vi "pipe writer.vi"() -> ()   [LabVIEW 2013, in "Unix Pipes.lvlib"]
uses:
  Unix Pipes.lvlib
  <vilib>/Platform/TimedLoop/XDataNode/timing_clust.ctl
  <vilib>/Platform/TimedLoop/XDataNode/nitl_modes.ctl
  <vilib>/Platform/TimedLoop/XDataNode/wakeup.ctl
  Classes/Unix Pipe Writer/Open Pipe (writer).vi
  Classes/Unix Pipe Writer/Close Pipe (writer).vi
  <vilib>/NI/NI Linux RT Utilities/VIs/Public/Time/Get Clock Time (timespec).vi
  <vilib>/platform/TimedLoop/XDataNode/XDataNode.xnode
  <vilib>/NI/NI Linux RT Utilities/Linux RT Utilities.lvlib
  Classes/Unix Pipe Writer/Unix Pipe Writer.lvclass
  <vilib>/Platform/TimedLoop/XDataNode/XDNodeRunTimeDep.lvlib
panel:
  out "pipe already exists?":bool
  in  "stop":bool
  out "time":cluster{"sec":u64, "nsec":u64}
  out "error out":errorcluster
  out "bytes written":i32
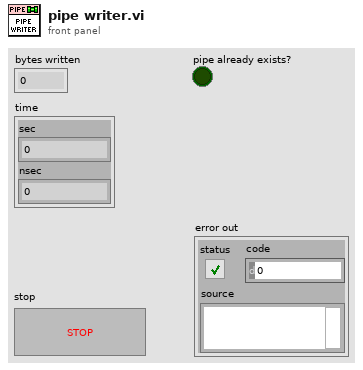
[diagram p1: front panel]
types:
  T1 = typedef "XDNodeRunTimeDep.lvlib/timing_clust.ctl" = cluster{"Expected End [f-1]":u64, "Actual End [f-1]":u64, "Finished Late? [f-1]":bool, "Expected End [i-1]":u64, "Actual End [i-1]":u64, "Finished Late? [i-1]":bool, "Expected Start [i]":u64, "Actual Start [i]":u64, "Expected Start [f]":u64, "Actual Start [f]":u64, "Source Name":string, "Structure Name":string, "Period":i64, "Deadline":i64, "Offset":i64, "Start":i64, "Priority":i32, "Timeout":i32, "Mode":T2, "Wakeup Reason":T3, "Error":errorcluster, "Source Type":string, "Secondary Source Type":string, "Global End Time":u64, "Global Start Time":u64, "Frame Duration":u64, "Iteration Duration":u64, "Assigned CPU":i32, "I/O Scan Engine Mode":u32}
  T2 = typedef "XDNodeRunTimeDep.lvlib/nitl_modes.ctl" = enum32{"No Change", "Process missed periods, maintain original phase", "Discard missed periods, maintain original phase", "Process missed periods, ignore original phase", "Discard missed periods, ignore original phase"}
  T3 = typedef "XDNodeRunTimeDep.lvlib/wakeup.ctl" = enum32{"Normal", "Aborted", "Asynchronous wakeup", "Timing source error", "Timed loop error", "Timeout"}
  T4 = enum16{"big-endian, network order", "native, host order", "little-endian"}
  T5 = cluster{"Stop":bool, "Time":cluster{"sec":u64, "nsec":u64}}
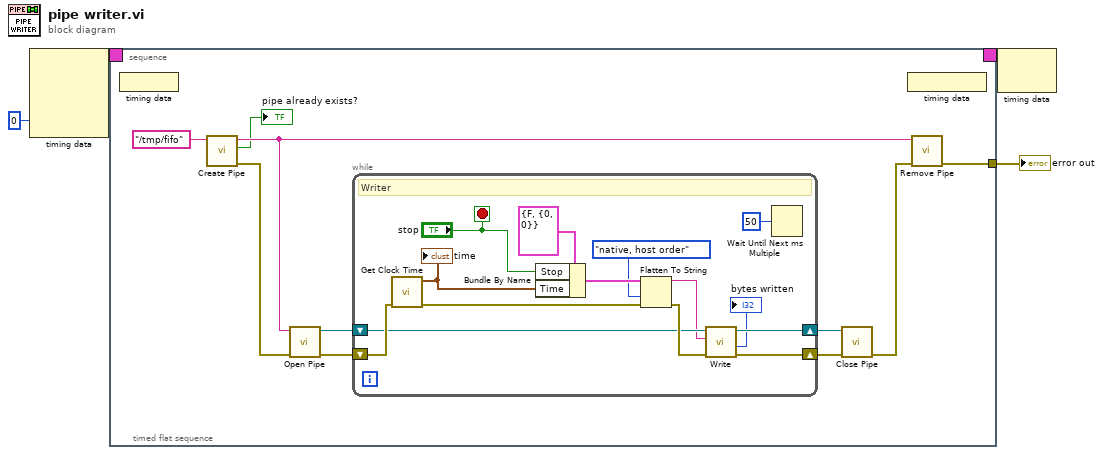
[diagram p0: block diagram]
diagram:
  n1 = node-c288(0 ("Processor")) -> (w3:T1)  [unwired: 3 in]
  n2 = timed-sequence {
    timing: w3 -> [_]
    timing-out: [_] -> w2
    tunnel: [w5] -> w4
    n3 = timed-flat-sequence {
      tunnel: [w13] -> w5
      n4 = node-c288() -> ()  [unwired: 1 in]
      n5 = call "Create Pipe.vi"("pathname in"="/tmp/fifo") -> ("error out"=w14:errorcluster, "pipe already exists?"=→"pipe already exists?":bool, "pathname out"=w7:string)  [unwired: 8 in]
      n6 = call-poly "Open Pipe.vi"("error in (no error)"=w14, "pathname in"=w7) -> ("error out"=w8:errorcluster, "pipe writer out"=w12:refnum<data-value>)  [unwired: 8 in]
      n7 = while {
        shift-right: [w28] -> w11
        shift-left: w12 -> [w17]
        shift-right: [w27] -> w10
        shift-left: w8 -> [w25]
        stop <- "stop" stop-if-true
        # "Writer"
        n8 = call-poly <vilib>:"Get Clock Time.vi"("error in (no error)"=w25) -> ("error out"=w20:errorcluster, "timespec"=w18:cluster{"sec":u64, "nsec":u64})  [unwired: 9 in]
        "time" <- w18
        n9 = Bundle By Name(cluster=T5 {"Stop"=FALSE, "Time"={"sec"=0, "nsec"=0}}, "Stop"="stop", "Time"=w18) -> (w22:T5)
        n10 = Flatten To String(anything=w22, byte order (0:big-endian, network order)=T4."native, host order", error in (no error)=w20) -> (data string=w16:string, error out=w21:errorcluster)  [unwired: 1 in, 1 out]
        n11 = call "Write.vi"("error in (no error)"=w21, "data"=w16, "pipe writer in"=w17) -> ("error out"=w27:errorcluster, "bytes written"=→"bytes written":i32, "pipe writer out"=w28:refnum<data-value>)  [unwired: 6 in]
        n12 = Wait Until Next ms Multiple(millisecond multiple=u32 50 ("wait")) -> ()  [unwired: 1 out]
      }
      n13 = call-poly "Close Pipe.vi"("error in (no error)"=w10, "pipe in"=w11) -> ("error out"=w9:errorcluster)  [unwired: 8 in, 1 out]
      n14 = node-c288() -> ()  [unwired: 1 out]
      n15 = call "Remove Pipe.vi"("error in (no error)"=w9, "pathname in"=w7) -> ("error out"=w13:errorcluster)  [unwired: 9 in]
    }
  }
  "error out" <- w4
  n16 = node-c288(w2) -> ()  [unwired: 1 out]
